vi "Error to String.vi"(10 "error in (no error)":errorcluster) -> (2 "String out":string)   [LabVIEW 2013]
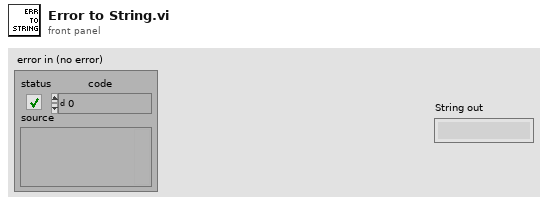
[diagram p1: front panel]
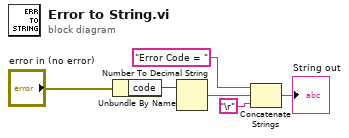
[diagram p0: block diagram]
diagram:
  n1 = Unbundle By Name("error in (no error)") -> ("code"=w5:i32)
  n2 = Number To Decimal String(number=w5) -> (decimal integer string=w4:string)  [unwired: 1 in]
  n3 = Concatenate Strings("Error Code = ", w4, "\r") -> (→"String out":string)
